vi "Seg2_discharging_setting.vi"(0 "VISA Refnum in":refnum<visa-resource-name>, 1 "N":string, 3 "Data Log Period (0.1 s)":dbl=1.0 format="%#_13g", 5 "Discharg current Limit":dbl=-0.1 format="%#_13f", 7 "Dischage - Range":T1(ring), 9 "Value":string, 11 "error in (no error)":errorcluster, 12 "Number of cycles":i32, 14 "Log?":bool) -> (4 "VISA Refnum out":refnum<visa-resource-name>, 6 "String out":string, 10 "File Name Out":string, 15 "error out":errorcluster)   [LabVIEW 2015]
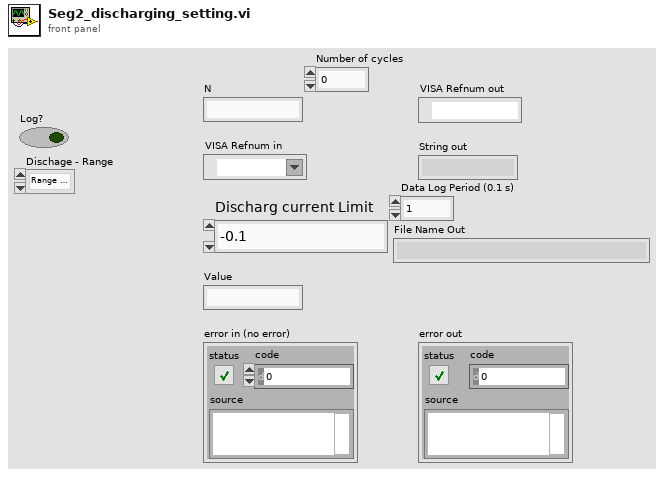
[diagram p1: front panel]
types:
  T1 = enum16{"Range 1 - 306mA", "Range 2 - 1.02 A", "Range 3 -  3.06"}
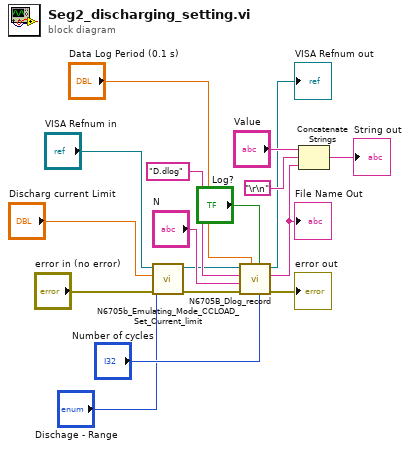
[diagram p0: block diagram]
diagram:
  n1 = call "N6705b_Emulating_Mode_CCLOAD_Set_Current_limit.vi"("error in (no error)"="error in (no error)", "Dischage - Range"="Dischage - Range", "Limit (0.0 amps)"="Discharg current Limit", "VISA Refnum in"="VISA Refnum in") -> ("error out"=w9:errorcluster, "VISA Refnum out"=w8:refnum<visa-resource-name>)  [unwired: 6 in]
  n2 = call "N6705B_Dlog_record.vi"("Number of cycles"="Number of cycles", "Log?"="Log?", "Data Log Period (0.1 s)"="Data Log Period (0.1 s)", "error in (no error)"=w9, "N"="N", "Data Log File Path (data1.dlog)"="D.dlog", "VISA resource name"=w8) -> ("error out"=→"error out":errorcluster, "File Name Out"=w16:string, "VISA resource name out"=→"VISA Refnum out":refnum<visa-resource-name>)  [unwired: 2 in]
  "File Name Out" <- w16
  n3 = Concatenate Strings("Value", "\r\n", w16) -> (→"String out":string)
